vi "StringParser.vi"(1 "String":string) -> (0 "array":string[](array[string]))   [LabVIEW 2014]
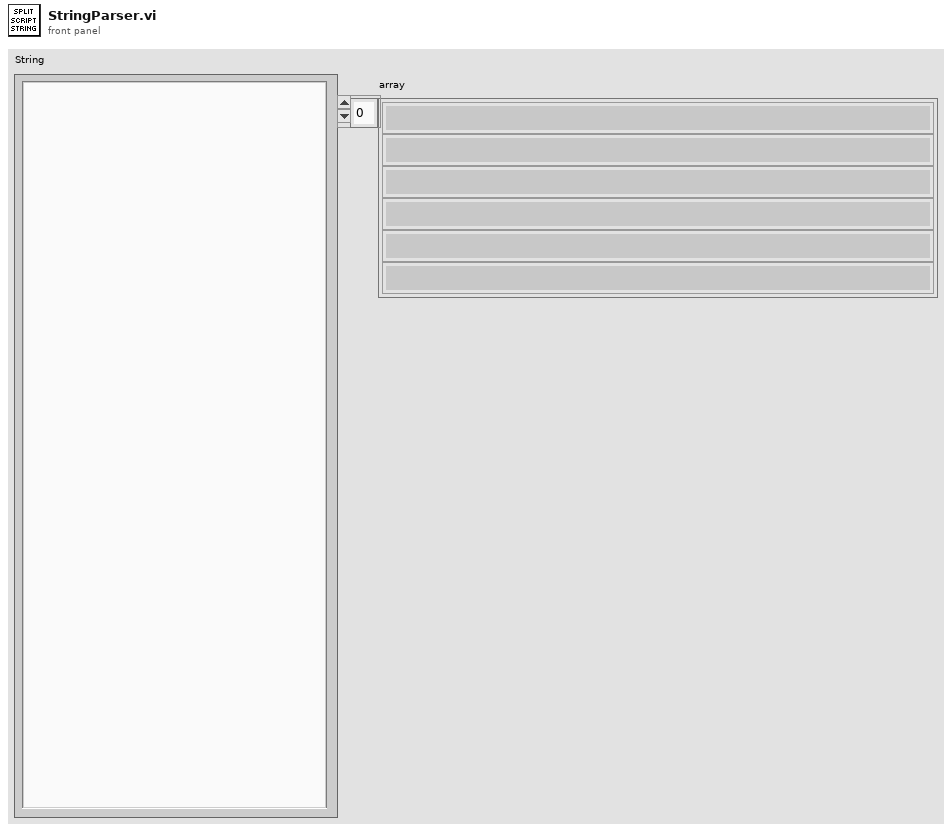
[diagram p1: front panel]
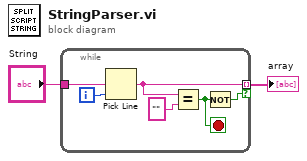
[diagram p0: block diagram]
diagram:
  n1 = while {
    tunnel: "String" -> [w8]
    tunnel: [w6] -> w1 mode=indexing if=w4
    i -> [w7]
    stop <- w3 stop-if-true
    n2 = Pick Line(multi-line string=w8, line index=w7) -> (output string=w6:string)  [unwired: 1 in]
    n3 = Equal?(x=w6, y="") -> (x = y?=w3:bool)
    n4 = Not(x=w3) -> (.not. x?=w4:bool)
  }
  "array" <- w1
